vi "Select_a_Channel.vi"(6 "Mode":T1(ring), 7 "Extra channel names":string[](array[string]), 8 "Data Filename":path) -> (0 "Current Values":string[](array[string]), 1 "Channel Values":string[](array[string]), 2 "Selected Channel Names":string[](array[string]), 3 "Data Filename Out":path)   [LabVIEW 2016]
uses:
  ADAM Client/Sub VIs/ADAM Controls/Channel_names.ctl
  ADAM Client/Sub VIs/ADAM Controls/Calib_type_ADAM.ctl
panel:
  in  "Tolerance":dbl=1.0 format="%.4f"
  in  "OK":bool
  in  "Search String":string
  in  "Listbox":i32[](listbox)
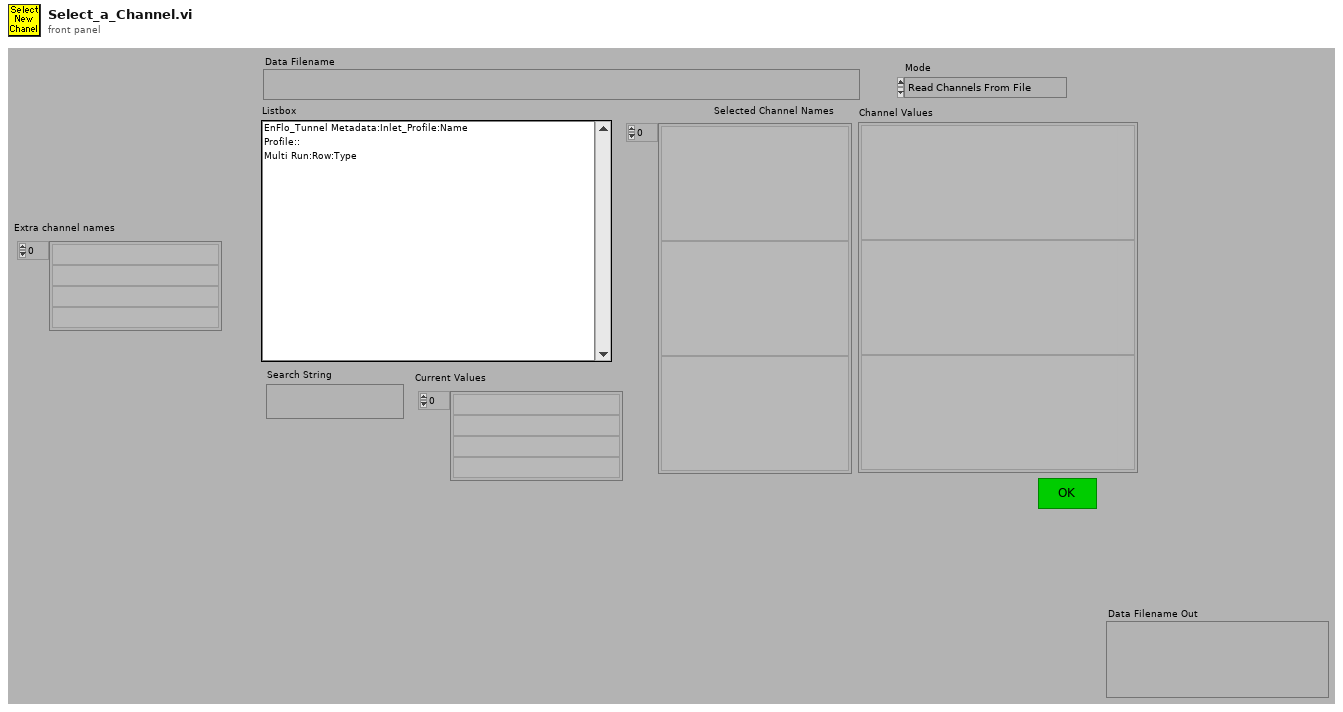
[diagram p1: front panel]
types:
  T1 = enum16{"Read Channels From File", "Read Channels from Server"}
  T2 = typedef "Channel_names.ctl" = enum16{"Active Only", "Active + Off", "All Channels"}
  T3 = enum32{"existing file", "new file", "new or existing file", "existing dir", "new dir", "new or existing dir", "existing file (use LLBs)", "new file (use LLBs)", "new or existing file (use LLBs)", "new or existing file or directory (use LLBs)"}
  T4 = typedef "Ch_description_ADAM.ctl" = cluster{"Ch Name":string, "Type":T5, "Function":T6, "Ch State":T7, "Calibration type":T8, "A":dbl, "B":dbl, "C":dbl, "D":dbl, "Comments":string, "Address":T9, "String":string, "Duty":u16}
  T5 = typedef "Module_type_ADAM.ctl" = string
  T6 = typedef "Function_ADAM.ctl" = enum16{"Analogue Input", "Digital Input", "Event counter", "Event rate", "Analogue Output", "Digital Output", "Relay Output"}
  T7 = typedef "Channel_State.ctl" = enum16{"On", "Off", "Always On", "Always Off"}
  T8 = typedef "Calib_type_ADAM.ctl" = string
  T9 = typedef "Address.ctl" = cluster{"Main":i32, "Ch.":i32, "Sub":i32, "Port Name":string}
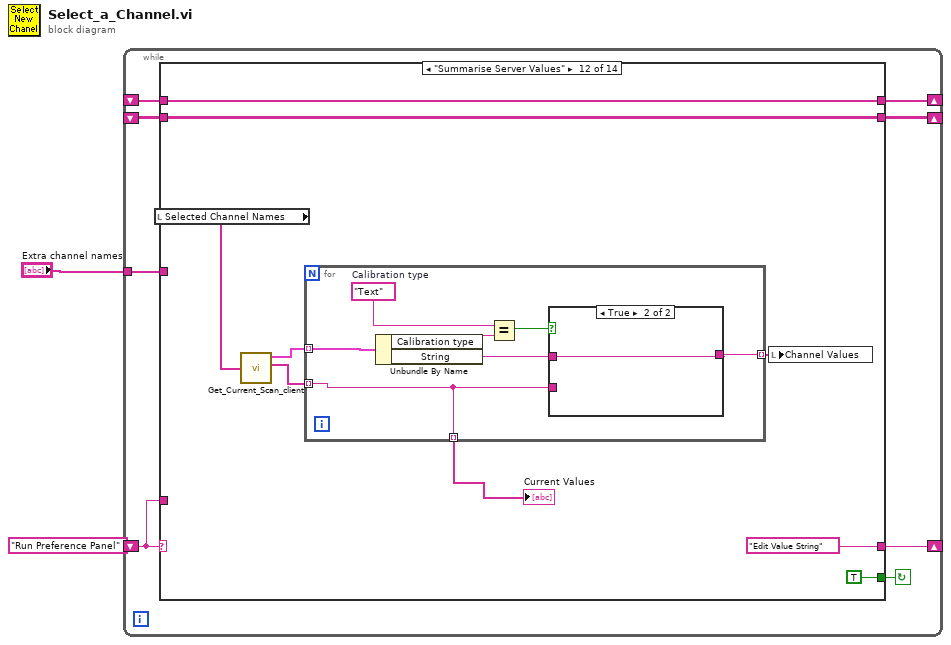
[diagram p0: block diagram]
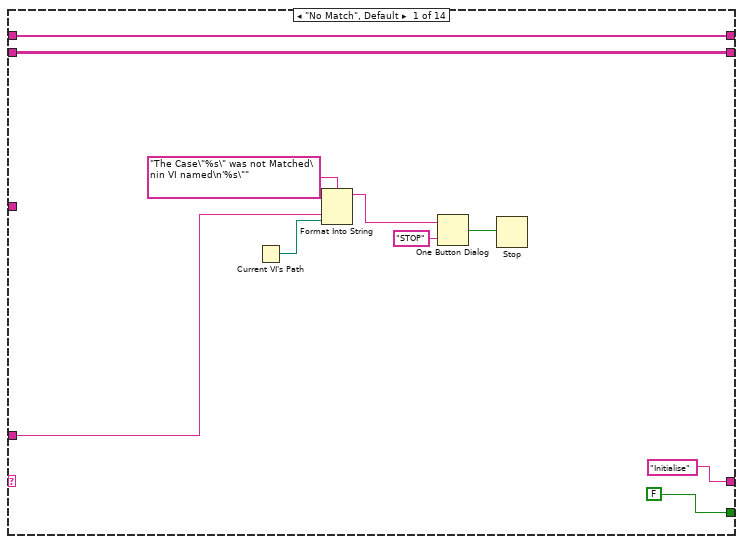
[diagram p2: hidden frame]
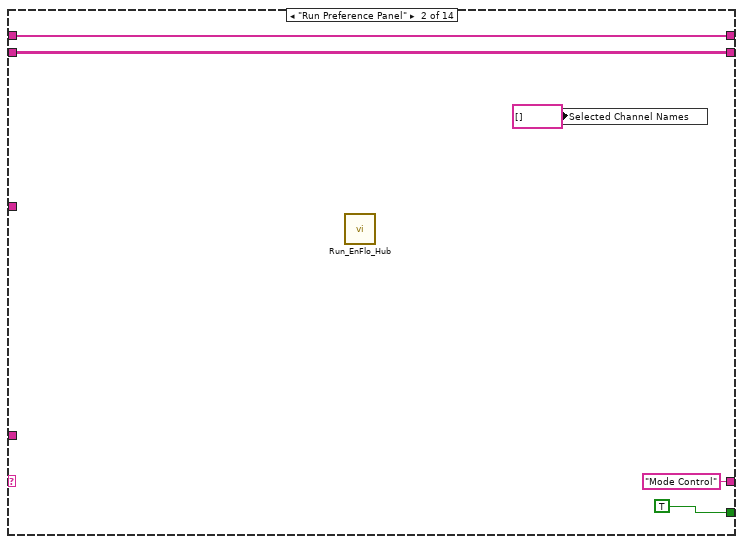
[diagram p3: hidden frame]
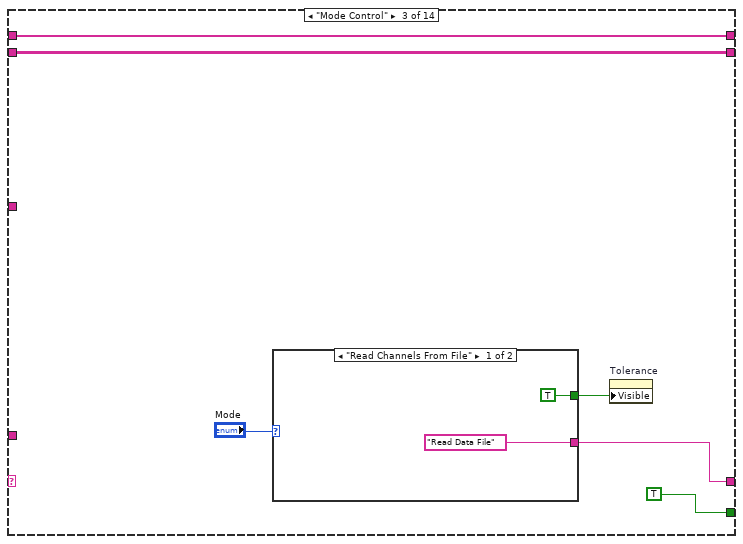
[diagram p4: hidden frame]
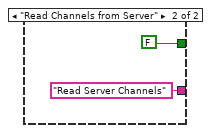
[diagram p5: hidden frame]
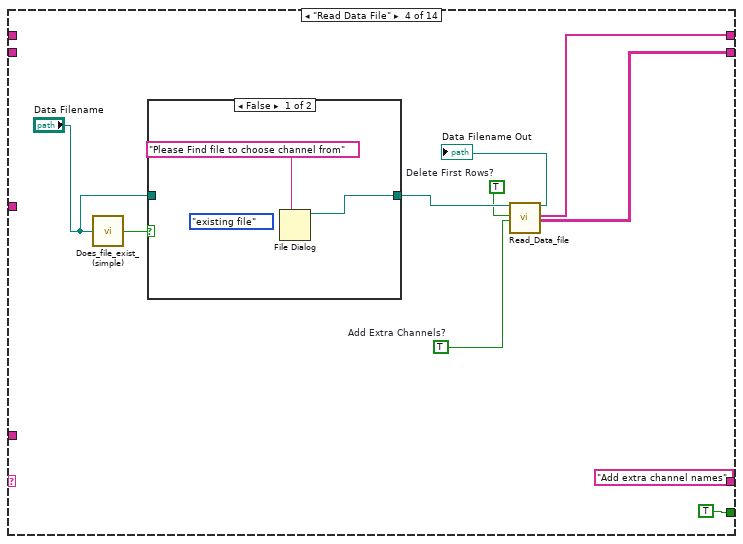
[diagram p6: hidden frame]
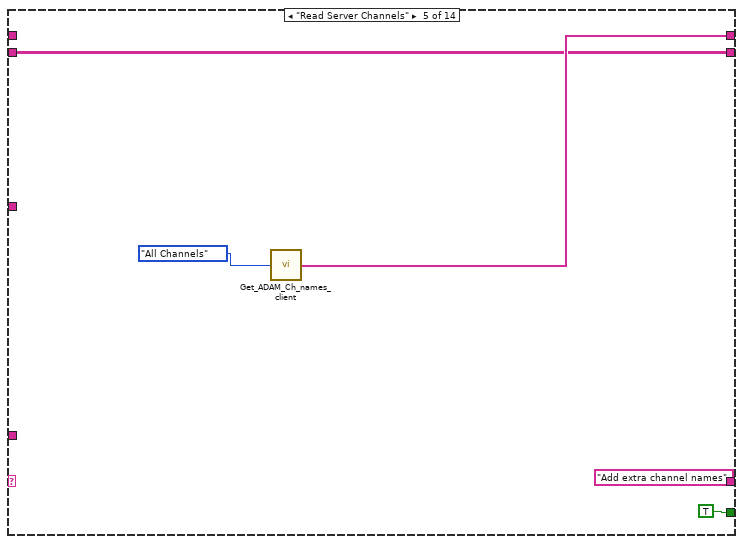
[diagram p8: hidden frame]
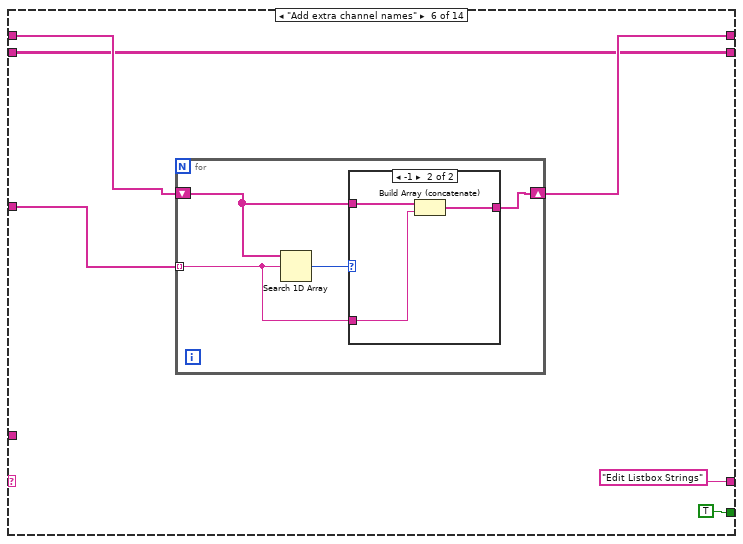
[diagram p9: hidden frame]
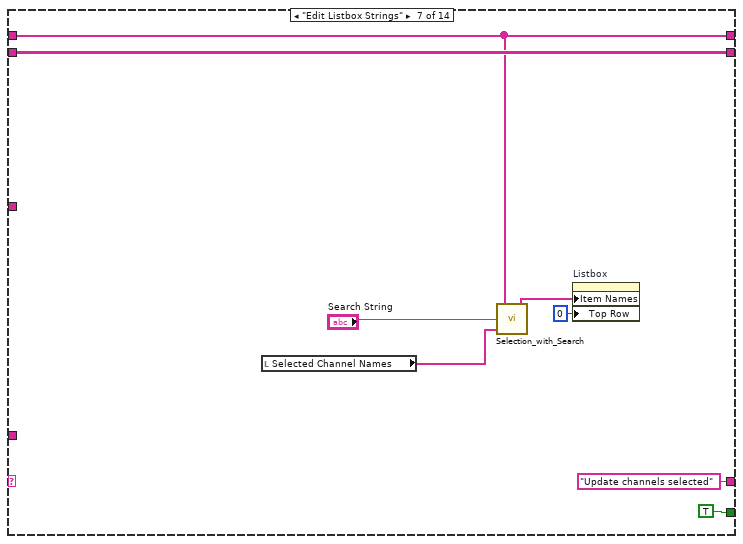
[diagram p11: hidden frame]
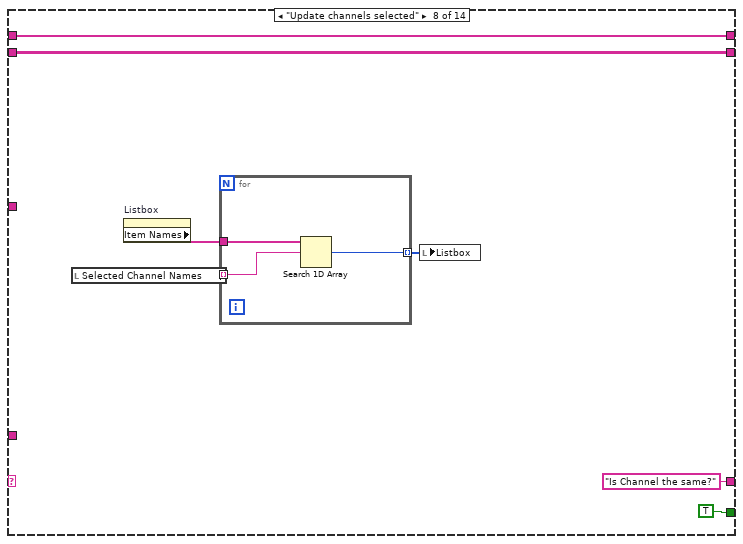
[diagram p12: hidden frame]
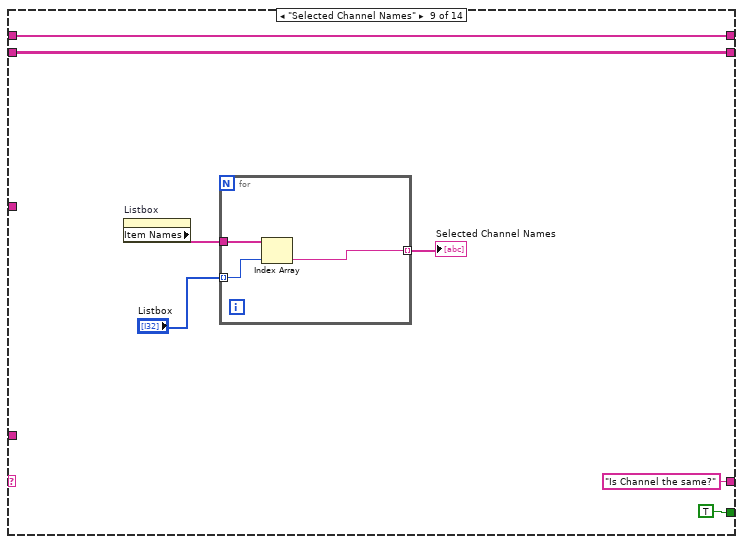
[diagram p13: hidden frame]
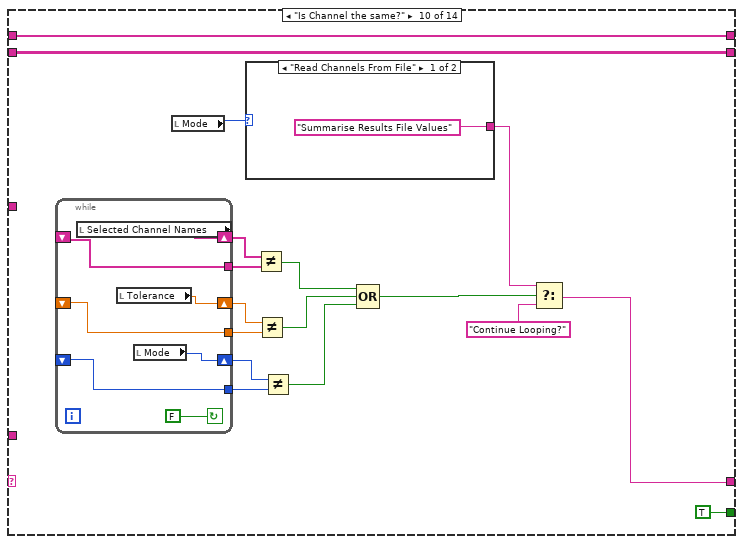
[diagram p14: hidden frame]
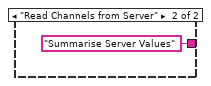
[diagram p15: hidden frame]
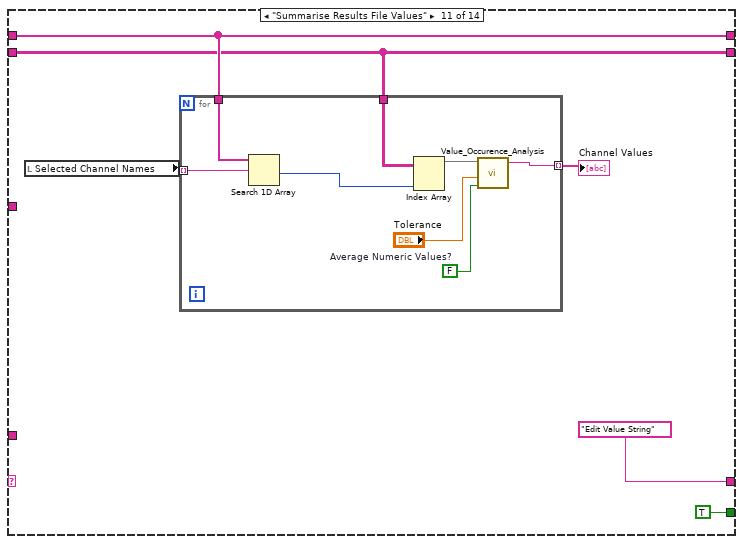
[diagram p16: hidden frame]
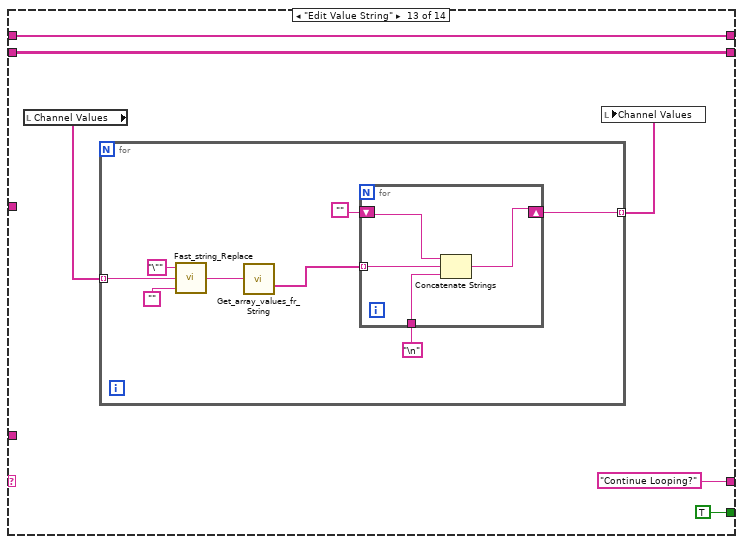
[diagram p18: hidden frame]
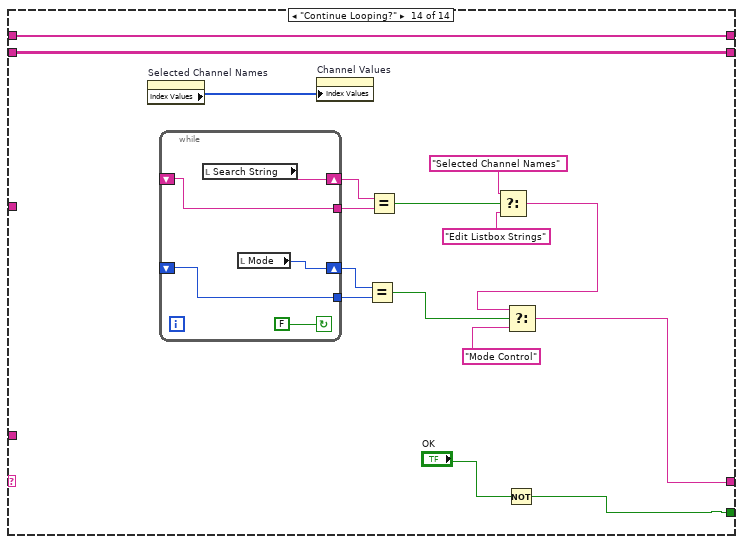
[diagram p19: hidden frame]
diagram:
  n1 = while {
    shift-left: _ -> [w4]
    shift-right: [w6] -> _
    shift-left: _ -> [w5]
    shift-right: [w7] -> _
    shift-left: "Run Preference Panel" -> [w8]
    shift-right: [w9] -> _
    tunnel: "Extra channel names" -> [w3]
    stop <- w10 continue-if-true
    n2 = case shown="\"Summarise Server Values\"" w8 {
      tunnel: [FALSE TRUE TRUE TRUE TRUE TRUE TRUE TRUE TRUE TRUE TRUE TRUE TRUE w184] -> w10
      tunnel: ["Initialise" "Mode Control" w28 "Add extra channel names" "Add extra channel names" "Edit Listbox Strings" "Update channels selected" "Is Channel the same?" "Is Channel the same?" w107 "Edit Value String" "Edit Value String" "Continue Looping?" w179] -> w9
      tunnel: w8 -> [w15 _ _ _ _ _ _ _ _ _ _ _ _ _]
      tunnel: [w12 w24 w30 w43 w51 w55 w73 w80 w90 w110 w126 w141 w156 w187] -> w7
      tunnel: [w11 w23 w29 w42 w50 w54 w74 w81 w91 w111 w124 w142 w157 w186] -> w6
      tunnel: w5 -> [w12 w24 w30 _ _ w57 w73 w80 w90 w110 w126 w141 w156 w187]
      tunnel: w4 -> [w11 w23 w29 _ w50 w54 w74 w81 w91 w111 w124 w142 w157 w186]
      tunnel: w3 -> [_ _ _ _ _ w56 _ _ _ _ _ _ _ _]
      frame "No Match", Default {
        n3 = Current VI's Path() -> (path=w14:path)
        n4 = Format Into String(format string="The Case\"%s\" was not Matched\nin VI named\n'%s\"" ("Format String"), w15, w14) -> (resulting string=w18:string)  [unwired: 2 in, 1 out]
        n5 = One Button Dialog(message=w18, button name ("OK")="STOP") -> (true=w16:bool)
        n6 = Stop(stop? (T)=w16) -> ()
      }
      frame "Run Preference Panel" {
        n7 = call "Run_EnFlo_Hub.vi"() -> ()  [unwired: 1 in, 7 out]
        n8 = local write "Selected Channel Names"(string[] [] ("Selected Channel Names")) -> ()
      }
      frame "Mode Control" {
        n9 = case shown="\"Read Channels From File\"" "Mode" {
          tunnel: ["Read Data File" "Read Server Channels"] -> w28
          tunnel: [TRUE FALSE] -> w27
          frame "Read Channels From File" {
          }
          frame "Read Channels from Server" {
          }
        }
        n10 = property on="Tolerance" class="DigNum (strict)"("Visible"=w27) -> ()  [unwired: 2 in, 2 out]
      }
      frame "Read Data File" {
        w36 = TRUE  # Delete First Rows?
        w41 = TRUE  # Add Extra Channels?
        n11 = call "Does_file_exist_(simple).vi"("Pathname"="Data Filename") -> ("exists?"=w40:bool)
        n12 = case shown="False" w40 {
          tunnel: [w47 w48] -> w38
          tunnel: "Data Filename" -> [_ w48]
          frame False {
            (unwired) T3."existing file" ("select mode (2)")
            n13 = File Dialog(7:"Please Find file to choose channel from" ("prompt")) -> (3:w47:path)  [unwired: 1 in, 8 out]
          }
          frame True {
          }
        }
        n14 = call "Read_Data_file.vi"("Results file"=w38, "Delete First Rows?"=w36, "Add Extra Channels?"=w41) -> ("Results file Out"=→"Data Filename Out":path, "Ch names Out"=w43:string[], "Channel Values Out"=w42:string[][])  [unwired: 4 in, 10 out]
      }
      frame "Read Server Channels" {
        n15 = call "Get_ADAM_Ch_names_client.vi"("Channel names set"=Channel_names."All Channels") -> ("Ch names"=w51:string[])
      }
      frame "Add extra channel names" {
        n16 = for {
          shift-right: [w61] -> w55
          shift-left: w57 -> [w62]
          tunnel: w56 -> [w60] mode=indexing
          n17 = Search 1D Array(1D array=w62, element=w60) -> (index of element=w63:i32)  [unwired: 1 out]
          n18 = case shown="-1" w63 {
            tunnel: w62 -> [w64 w67]
            tunnel: [w64 w66] -> w61
            tunnel: w60 -> [_ w65]
            frame 0, Default {
            }
            frame -1 {
              n19 = Build Array (concatenate)(w67, w65) -> (w66:string[])
            }
          }
        }
      }
      frame "Edit Listbox Strings" {
        n20 = local read "Selected Channel Names"() -> (w69:string[])
        n21 = call "Selection_with_Search.vi"("Selected Channel Names"=w69, "Search String"="Search String", "All Channel Names"=w73) -> ("Item Names"=w70:string[])
        n22 = property on="Listbox" class="LstBox (strict)"("Item Names"=w70, "Top Row"=0) -> ()  [unwired: 2 in, 2 out]
      }
      frame "Update channels selected" {
        n23 = local read "Selected Channel Names"() -> (w77:string[])
        n24 = property on="Listbox" class="LstBox (strict)"() -> ("Item Names"=w78:string[])  [unwired: 2 in, 2 out]
        n25 = for {
          tunnel: w78 -> [w85]
          tunnel: w77 -> [w84] mode=indexing
          tunnel: [w83] -> w76 mode=indexing
          n26 = Search 1D Array(1D array=w85, element=w84) -> (index of element=w83:i32)  [unwired: 1 out]
        }
        n27 = local write "Listbox"(w76) -> ()
      }
      frame "Selected Channel Names" {
        n28 = property on="Listbox" class="LstBox (strict)"() -> ("Item Names"=w88:string[])  [unwired: 2 in, 2 out]
        n29 = for {
          tunnel: w88 -> [w95]
          tunnel: "Listbox" -> [w94] mode=indexing
          tunnel: [w93] -> w86 mode=indexing
          n30 = Index Array(array=w95, index=w94) -> (element=w93:string)
        }
        "Selected Channel Names" <- w86
      }
      frame "Is Channel the same?" {
        n31 = while {
          tunnel: [w115] -> w99
          shift-left: _ -> [w115]
          shift-right: [w114] -> w100
          tunnel: [w116] -> w106
          shift-left: _ -> [w116]
          shift-right: [w117] -> w105
          tunnel: [w118] -> w108
          shift-left: _ -> [w118]
          shift-right: [w119] -> w109
          stop <- FALSE continue-if-true
          n32 = local read "Selected Channel Names"() -> (w119:string[])
          n33 = local read "Tolerance"() -> (w117:dbl)
          n34 = local read "Mode"() -> (w114:T1)
        }
        n35 = local read "Mode"() -> (w101:T1)
        n36 = case shown="\"Read Channels From File\"" w101 {
          tunnel: ["Summarise Results File Values" "Summarise Server Values"] -> w97
          frame "Read Channels From File" {
          }
          frame "Read Channels from Server" {
          }
        }
        n37 = Not Equal?(x=w109, y=w108) -> (x != y?=w104:bool)
        n38 = Not Equal?(x=w105, y=w106) -> (x != y?=w103:bool)
        n39 = Not Equal?(x=w100, y=w99) -> (x != y?=w98:bool)
        n40 = Compound Arithmetic op=OR(w104, w103, w98) -> (w102:bool)
        n41 = Select(t=w97, s=w102, f="Continue Looping?") -> (s? t:f=w107:string)
      }
      frame "Summarise Results File Values" {
        n42 = local read "Selected Channel Names"() -> (w125:string[])
        n43 = for {
          tunnel: w126 -> [w135]
          tunnel: w125 -> [w134] mode=indexing
          tunnel: w124 -> [w132]
          tunnel: [w129] -> w122 mode=indexing
          w128 = FALSE  # Average Numeric Values?
          n44 = Search 1D Array(1D array=w135, element=w134) -> (index of element=w133:i32)  [unwired: 1 out]
          n45 = Index Array(array=w132, index (col)=w133) -> (element=w131:string[])  [unwired: 1 in]
          n46 = call "Value_Occurence_Analysis.vi"("Average Numeric Values?"=w128, "Tolerance"="Tolerance", "String Array"=w131) -> ("Output String"=w129:string)  [unwired: 1 in, 2 out]
        }
        "Channel Values" <- w122
      }
      frame "Summarise Server Values" {
        n47 = local read "Selected Channel Names"() -> (w140:string[])
        n48 = call "Get_Current_Scan_client.vi"("ADAM Ch Names"=w140) -> ("Ch Description Array"=w139:T4[], "String values"=w138:string[])  [unwired: 2 out]
        n49 = for {
          tunnel: w139 -> [w147] mode=indexing
          tunnel: w138 -> [w146] mode=indexing
          tunnel: [w148] -> w136 mode=indexing
          tunnel: [w146] -> w137 mode=indexing
          w145 = T8 "Text"  # Calibration type
          n50 = Unbundle By Name(w147) -> ("Calibration type"=w151:T8, "String"=w149:string)
          n51 = Equal?(x=w145, y=w151) -> (x = y?=w150:bool)
          n52 = case shown="True" w150 {
            tunnel: [w152 w153] -> w148
            tunnel: w149 -> [_ w153]
            tunnel: w146 -> [w152 _]
            frame False {
            }
            frame True {
            }
          }
        }
        "Current Values" <- w137
        n53 = local write "Channel Values"(w136) -> ()
      }
      frame "Edit Value String" {
        n54 = local read "Channel Values"() -> (w155:string[])
        n55 = for {
          tunnel: w155 -> [w161] mode=indexing
          tunnel: [w160] -> w154 mode=indexing
          n56 = call "Fast_string_Replace.vi"("Replace match with:"="", "Input String"=w161, "regular expression"="\"") -> ("Output String"=w162:string)  [unwired: 2 out]
          n57 = call "Get_array_values_fr_String.vi"("String Value"=w162) -> ("String array"=w167:string[])  [unwired: 1 out]
          n58 = for {
            shift-right: [w168] -> w160
            shift-left: "" -> [w171]
            tunnel: w167 -> [w170] mode=indexing
            tunnel: "\n" -> [w169]
            n59 = Concatenate Strings(w171, w170, w169) -> (w168:string)
          }
        }
        n60 = local write "Channel Values"(w154) -> ()
      }
      frame "Continue Looping?" {
        n61 = property on="Selected Channel Names" class="Arr (strict)"() -> ("Index Values"=w172:u32[])  [unwired: 2 in, 2 out]
        n62 = while {
          tunnel: [w189] -> w178
          shift-left: _ -> [w189]
          shift-right: [w190] -> w177
          tunnel: [w192] -> w182
          shift-left: _ -> [w192]
          shift-right: [w191] -> w183
          stop <- FALSE continue-if-true
          n63 = local read "Search String"() -> (w190:string)
          n64 = local read "Mode"() -> (w191:T1)
        }
        n65 = property on="Channel Values" class="Arr (strict)"("Index Values"=w172) -> ()  [unwired: 2 in, 2 out]
        n66 = Equal?(x=w183, y=w182) -> (x = y?=w181:bool)
        n67 = Equal?(x=w177, y=w178) -> (x = y?=w176:bool)
        n68 = Select(t="Selected Channel Names", s=w176, f="Edit Listbox Strings") -> (s? t:f=w173:string)
        n69 = Not(x="OK") -> (.not. x?=w184:bool)
        n70 = Select(t=w173, s=w181, f="Mode Control") -> (s? t:f=w179:string)
      }
    }
  }
